vi "RemoveObject.vi"(8 "error in (no error)":errorcluster, 9 "Ancestor":string, 10 "Name":string, 11 "reference in":refnum<class "ViPER.lvclass">) -> (0 "error out":errorcluster, 3 "reference out":refnum<class "ViPER.lvclass">)   [LabVIEW 2022 SP3, in "ViPER.lvlib" / "ViPER.lvclass"]
doc: "### BSD License (http://www.opensource.org/licenses/bsd-license.php) Begin ###\n\nCopyright (c) 2018 Kurt Friday www.medulla.net\n\nAll rights reserved.\n\nRedistribution and use in source and binary forms, with or without\nmodification, are permitted provided that the following conditions are met:\n\n * Redistributions of source code must retain the above copyright\n notice, this list of conditions and the following disclaimer.\n\n * Redistributions in binary form must reproduce the above copyright\n notice, this list of conditions and the following disclaimer in the\n documentation and/or other materials provided with the distribution.\n\n * Neither the name of the <organization> nor the\n names of its contributors may be used to endorse or promote products\n derived from this software without specific prior written permission.\n\nTHIS SOFTWARE IS PROVIDED BY THE COPYRIGHT HOLDERS AND CONTRIBUTORS \"AS IS\" AND\nANY EXPRESS OR IMPLIED WARRANTIES, INCLUDING, BUT NOT LIMITED TO, THE IMPLIED\nWARRANTIES OF MERCHANTABILITY AND FITNESS FOR A PARTICULAR PURPOSE ARE\nDISCLAIMED. IN NO EVENT SHALL <COPYRIGHT HOLDER> BE LIABLE FOR ANY\nDIRECT, INDIRECT, INCIDENTAL, SPECIAL, EXEMPLARY, OR CONSEQUENTIAL DAMAGES\n(INCLUDING, BUT NOT LIMITED TO, PROCUREMENT OF SUBSTITUTE GOODS OR SERVICES;\nLOSS OF USE, DATA, OR PROFITS; OR BUSINESS INTERRUPTION) HOWEVER CAUSED AND\nON ANY THEORY OF LIABILITY, WHETHER IN CONTRACT, STRICT LIABILITY, OR TORT\n(INCLUDING NEGLIGENCE OR OTHERWISE) ARISING IN ANY WAY OUT OF THE USE OF THIS\nSOFTWARE, EVEN IF ADVISED OF THE POSSIBILITY OF SUCH DAMAGE."
uses:
  ViPER.lvclass
panel:
  # "### BSD License (http://www.opensource.org/licenses/bsd-license.php) Begin ###\n\nCopyright (c) 2018  Kurt Friday www.medulla.net\n\nAll rights reserved.\n\nRedistribution and use in source and binary forms, with or without\nmodification, are permitted provided that the following conditions are met:\n\n    * Redistributions of source code must retain the above copyright\n      notice, this list of conditions and the following disclaimer.\n\n    * Redistributions in binary form must reproduce the above copyright\n      notice, this list of conditions and the following disclaimer in the\n      documentation and/or other materials provided with the distribution.\n\n    * Neither the name of the <organization> nor the\n      names of its contributors may be used to endorse or promote products\n      derived from this software without specific prior written permission.\n\nTHIS SOFTWARE IS PROVIDED BY THE COPYRIGHT HOLDERS AND CONTRIBUTORS \"AS IS\" AND\nANY EXPRESS OR IMPLIED WARRANTIES, INCLUDING, BUT NOT LIMITED TO, THE IMPLIED\nWARRANTIES OF MERCHANTABILITY AND FITNESS FOR A PARTICULAR PURPOSE ARE\nDISCLAIMED. IN NO EVENT SHALL <COPYRIGHT HOLDER> BE LIABLE FOR ANY\nDIRECT, INDIRECT, INCIDENTAL, SPECIAL, EXEMPLARY, OR CONSEQUENTIAL DAMAGES\n(INCLUDING, BUT NOT LIMITED TO, PROCUREMENT OF SUBSTITUTE GOODS OR SERVICES;\nLOSS OF USE, DATA, OR PROFITS; OR BUSINESS INTERRUPTION) HOWEVER CAUSED AND\nON ANY THEORY OF LIABILITY, WHETHER IN CONTRACT, STRICT LIABILITY, OR TORT\n(INCLUDING NEGLIGENCE OR OTHERWISE) ARISING IN ANY WAY OUT OF THE USE OF THIS\nSOFTWARE, EVEN IF ADVISED OF THE POSSIBILITY OF SUCH DAMAGE."
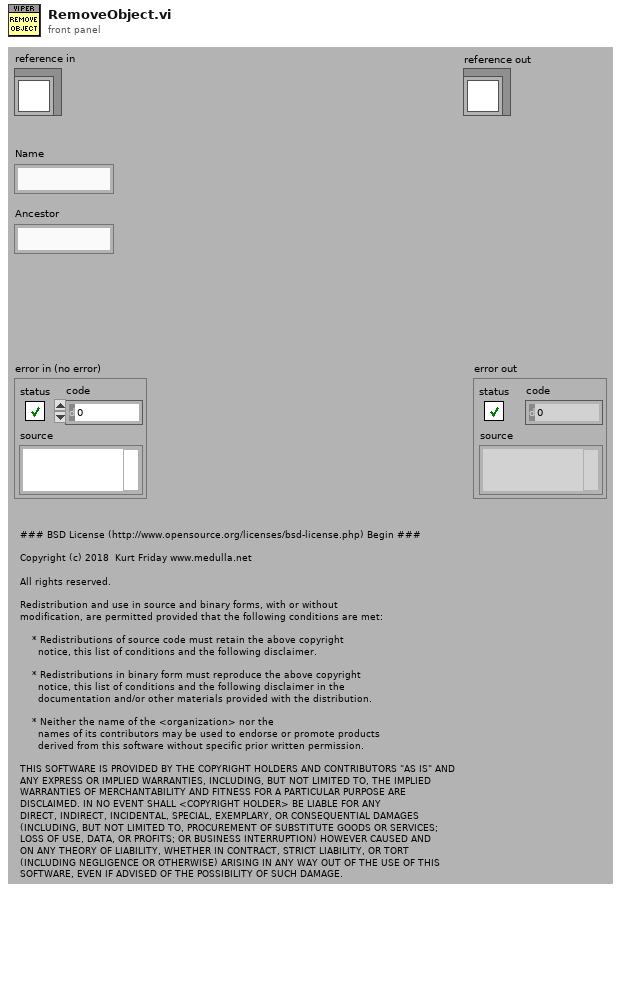
[diagram p1: front panel]
types:
  T1 = typedef "ViPER.lvlib/ViPER.lvclass/ObjectAttributes.ctl" = cluster{"Object":T2, "Ancestors":T4[], "Config":T5, "Init_OK":bool, "Hierachy":string[], "PPL?":bool[], "SFP_Open":bool[], "Config_SFP_Open":bool[], "SoftFP_event":refnum<user-event>[], "ConfigFP_event":refnum<user-event>[], "SoftFP_Shutdown_Notifier":refnum<notifier>[], "ConfigFP_Shutdown_Notifier":refnum<notifier>[]}
  T2 = typedef "ViPER.lvlib/ViPER.lvclass/ObjectDefinition.ctl" = cluster{"Name":string, "Ancestors":T3[]}
  T3 = typedef "ViPER.lvlib/ViPER.lvclass/Ancestor.ctl" = cluster{"Class":string, "Config":string, "Objects":string[]}
  T4 = typedef "ViPER.lvlib/ViPER.lvclass/ObjectLayers.ctl" = cluster{"Ancestor":string, "Objects":refnum<class "ViPER.lvclass">[], "Object_Names":string[], "Owned":bool[]}
  T5 = typedef "ViPER.lvlib/ViPER.lvclass/Config.ctl" = cluster{"default":string}
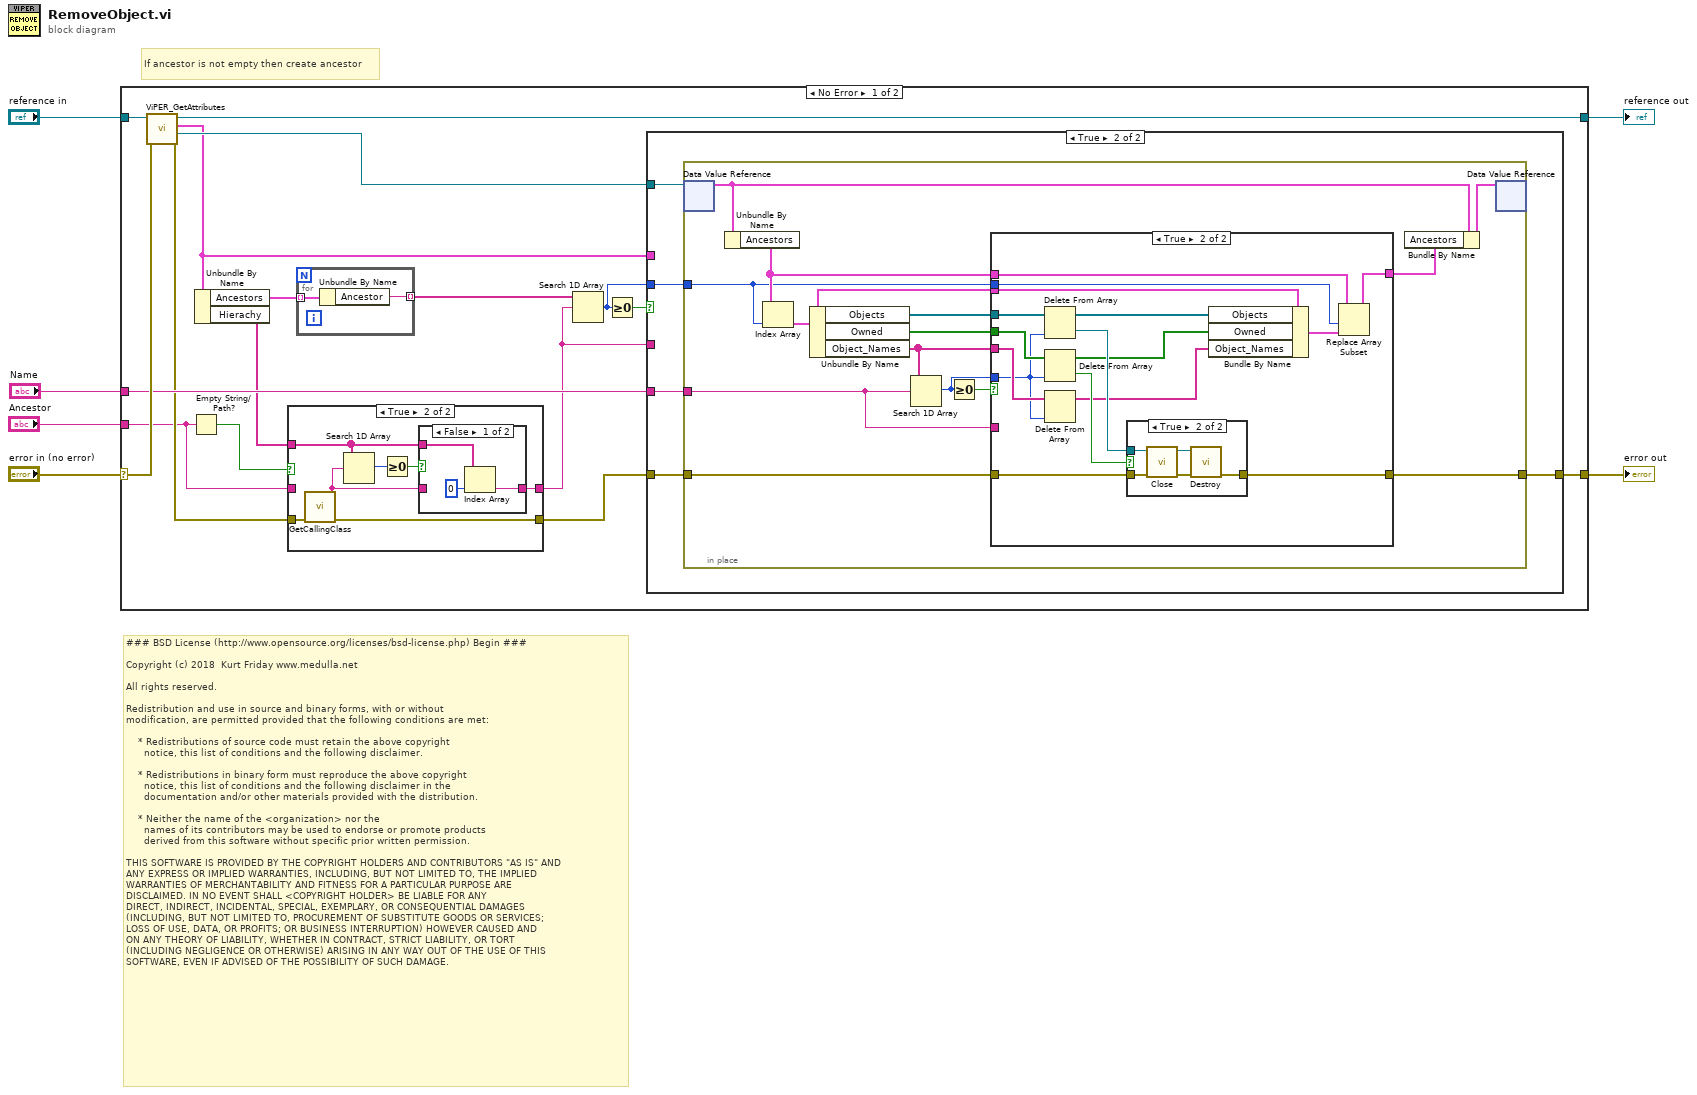
[diagram p0: block diagram]
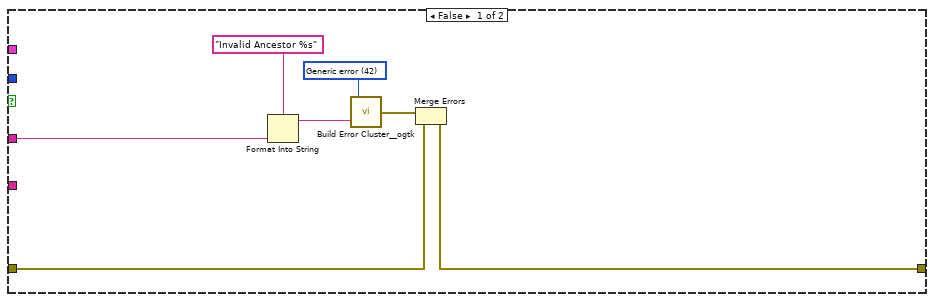
[diagram p4: hidden frame]
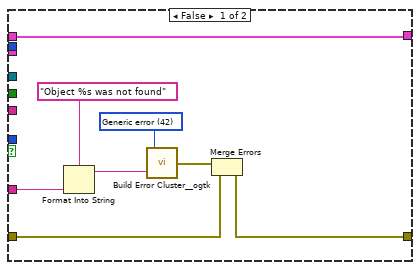
[diagram p5: hidden frame]
diagram:
  # "### BSD License (http://www.opensource.org/licenses/bsd-license.php) Begin ###\n\nCopyright (c) 2018  Kurt Friday www.medulla.net\n\nAll rights reserved.\n\nRedistribution and use in source and binary forms, with or without\nmodification, are permitted provided that the following conditions are met:\n\n    * Redistributions of source code must retain the above copyright\n      notice, this list of conditions and the following disclaimer.\n\n    * Redistributions in binary form must reproduce the above copyright\n      notice, this list of conditions and the following disclaimer in the\n      documentation and/or other materials provided with the distribution.\n\n    * Neither the name of the <organization> nor the\n      names of its contributors may be used to endorse or promote products\n      derived from this software without specific prior written permission.\n\nTHIS SOFTWARE IS PROVIDED BY THE COPYRIGHT HOLDERS AND CONTRIBUTORS \"AS IS\" AND\nANY EXPRESS OR IMPLIED WARRANTIES, INCLUDING, BUT NOT LIMITED TO, THE IMPLIED\nWARRANTIES OF MERCHANTABILITY AND FITNESS FOR A PARTICULAR PURPOSE ARE\nDISCLAIMED. IN NO EVENT SHALL <COPYRIGHT HOLDER> BE LIABLE FOR ANY\nDIRECT, INDIRECT, INCIDENTAL, SPECIAL, EXEMPLARY, OR CONSEQUENTIAL DAMAGES\n(INCLUDING, BUT NOT LIMITED TO, PROCUREMENT OF SUBSTITUTE GOODS OR SERVICES;\nLOSS OF USE, DATA, OR PROFITS; OR BUSINESS INTERRUPTION) HOWEVER CAUSED AND\nON ANY THEORY OF LIABILITY, WHETHER IN CONTRACT, STRICT LIABILITY, OR TORT\n(INCLUDING NEGLIGENCE OR OTHERWISE) ARISING IN ANY WAY OUT OF THE USE OF THIS\nSOFTWARE, EVEN IF ADVISED OF THE POSSIBILITY OF SUCH DAMAGE."
  # "If ancestor is not empty then create ancestor"
  n1 = case shown="No Error" "error in (no error)" {
    selector: "error in (no error)" -> [w21 w96]
    tunnel: [w17 w96] -> w5
    tunnel: [w22 w95] -> w3
    tunnel: "reference in" -> [w23 w95]
    tunnel: "Ancestor" -> [w9 _]
    tunnel: "Name" -> [w13 _]
    frame No Error {
      n2 = call "ViPER_GetAttributes.vi"("error in (no error)"=w21, "reference in"=w23) -> ("error out"=w12:errorcluster, "DataRef"=w15:refnum<data-value>, "Data"=w14:T1, "reference out"=w22:refnum<class "ViPER.lvclass">)  [unwired: 6 in]
      n3 = Empty String/Path?(string/path=w9) -> (empty?=w8:bool)
      n4 = Unbundle By Name(w14) -> ("Ancestors"=w20:T4[], "Hierachy"=w7:string[])
      n5 = case shown="True" w8 {
        tunnel: w12 -> [w24 w32]
        tunnel: [w24 w31] -> w11
        tunnel: [w25 w27] -> w10
        tunnel: w9 -> [w25 _]
        tunnel: w7 -> [_ w28]
        frame False {
        }
        frame True {
          n6 = call "GetCallingClass.vi"("error in (no error)"=w32) -> ("error out"=w31:errorcluster, "calling class"=w26:string)  [unwired: 9 in]
          n7 = Search 1D Array(1D array=w28, element=w26) -> (index of element=w30:i32)  [unwired: 1 in]
          n8 = Greater Or Equal To 0?(x=w30) -> (x >= 0?=w29:bool)
          n9 = case shown="False" w29 {
            tunnel: w28 -> [w35 _]
            tunnel: [w33 w36] -> w27
            tunnel: w26 -> [_ w36]
            frame False {
              n10 = Index Array(array=w35, index=0) -> (element=w33:string)
            }
            frame True {
            }
          }
        }
      }
      n11 = for {
        tunnel: w20 -> [w94] mode=indexing
        tunnel: [w93] -> w19 mode=indexing
        n12 = Unbundle By Name(w94) -> ("Ancestor"=w93:string)
      }
      n13 = Search 1D Array(1D array=w19, element=w10) -> (index of element=w16:i32)  [unwired: 1 in]
      n14 = Greater Or Equal To 0?(x=w16) -> (x >= 0?=w18:bool)
      n15 = case shown="True" w18 {
        tunnel: w11 -> [w39 w46]
        tunnel: [w38 w44] -> w17
        tunnel: w16 -> [_ w47]
        tunnel: w15 -> [_ w48]
        tunnel: w10 -> [w37 _]
        tunnel: w14 -> [_ _]
        tunnel: w13 -> [_ w45]
        frame False {
          w43 = 42 items=["No error", "Argument error", "Memory is full", "Out of zone", "End of file", "File already open", "Generic file I/O error", "File not found", "File permission error", "Disk is full", "Duplicate path", "Too many files open", "System feature not enabled", "Resource file not found", "Cannot add resource", "Resource not found", "Image not found", "Image memory error", "Pen does not exist", "Config type invalid", "Config token not found", "Config parse error", "Config memory error", "Bad external code format", "Bad external code offset", "External code not present", "Null window", "Destroy window error", "Null menu", "Print aborted", "Bad print record", "Print driver error", "Windows error during printing", "Memory error during printing", "Print dialog error", "Generic print error", "Invalid device refnum", "Device not found", "Device parameter error", "Device unit error", "Cannot open device", "Device call aborted", "Generic error", "Cancelled by user", "Object ID too low", "Object ID too high", "Object not in heap", "Unknown heap", "Unknown object (invalid DefProc)", "Unknown object (DefProc not in table)", "Message out of range", "Invalid (null) method", "Unknown message", "Manager call not supported", "Bad address", "Network operation in progress", "Network operation timed out", "Connection is busy", "Network attribute not supported", "Network error", "Address in use", "System out of memory", "Connection aborted", "Connection refused", "Not connected", "Already connected", "Connection closed", "Initialization error (interapplication manager)", "Bad occurrence", "Wait on unbound occurrence handler", "Occurrence queue overflow", "Datalog type conflict", "Unused", "Unrecognized type (interapplication manager)", "Memory corrupt", "Failed to make temporary DLL", "Old CIN version", "Drag socket not found", "Failed to load drop-object", "Failed to register OLE object", "Failed to release OLE object", "Format specifier type mismatch", "Unknown format specifier", "Too few format specifiers", "Too many format specifiers", "Scan failed", "Newer CIN version", "Error converting to variant", "Runtime menu error", "Password tampered", "Variant attribute not found", "Incompatible variant data type", "Event data is not available", "Event Store is not present", "Occurrence is not found", "Event Queue is not created", "Event info is not available", "Refnum passed is NULL", "Error retrieving Class GUID", "Error retrieving CoClass GUID", "Error retrieving TypeLib GUID.", "Bad built application magic bytes.", "Specific driver is different from the specific driver associated with the Logical Name.", "There is no session opened to the class driver.", "Max Error", "MAX - Error with config objects", "MAX - Error loading configuration", "MAX - Group not supported"]
          n16 = Format Into String(format string="Invalid Ancestor %s", w37) -> (resulting string=w40:string)  [unwired: 2 in, 1 out]
          n17 = call <userlib>:"Build Error Cluster__ogtk.vi"("String to Prepend to source (\"\")"=w40, "code"=w43) -> ("error out"=w42:errorcluster)
          n18 = Merge Errors(w42, w39) -> (w38:errorcluster)
        }
        frame True {
          n19 = in-place {
            in-place-border: w47 -> [w53]
            in-place-border: w46 -> [w51]
            in-place-border: w45 -> [w49]
            in-place-border: [w50] -> w44
            n20 = in-place-dvr #1(w48) -> (w61:T1)  [unwired: 1 out]
            n21 = Unbundle By Name(w61) -> ("Ancestors"=w60:T4[])
            n22 = Index Array(array=w60, index=w53) -> (element=w59:T4)
            n23 = Unbundle By Name(w59) -> ("Objects"=w54:refnum<class "ViPER.lvclass">[], "Owned"=w55:bool[], "Object_Names"=w56:string[])
            n24 = Search 1D Array(1D array=w56, element=w49) -> (index of element=w52:i32)  [unwired: 1 in]
            n25 = Greater Or Equal To 0?(x=w52) -> (x >= 0?=w57:bool)
            n26 = case shown="True" w57 {
              tunnel: w60 -> [w70 w86]
              tunnel: w59 -> [_ w85]
              tunnel: [w70 w83] -> w58
              tunnel: w56 -> [_ w78]
              tunnel: w55 -> [_ w79]
              tunnel: w54 -> [_ w81]
              tunnel: w53 -> [_ w82]
              tunnel: w52 -> [_ w77]
              tunnel: w51 -> [w67 w75]
              tunnel: [w66 w73] -> w50
              tunnel: w49 -> [w65 _]
              frame False {
                w69 = 42 items=["No error", "Argument error", "Memory is full", "Out of zone", "End of file", "File already open", "Generic file I/O error", "File not found", "File permission error", "Disk is full", "Duplicate path", "Too many files open", "System feature not enabled", "Resource file not found", "Cannot add resource", "Resource not found", "Image not found", "Image memory error", "Pen does not exist", "Config type invalid", "Config token not found", "Config parse error", "Config memory error", "Bad external code format", "Bad external code offset", "External code not present", "Null window", "Destroy window error", "Null menu", "Print aborted", "Bad print record", "Print driver error", "Windows error during printing", "Memory error during printing", "Print dialog error", "Generic print error", "Invalid device refnum", "Device not found", "Device parameter error", "Device unit error", "Cannot open device", "Device call aborted", "Generic error", "Cancelled by user", "Object ID too low", "Object ID too high", "Object not in heap", "Unknown heap", "Unknown object (invalid DefProc)", "Unknown object (DefProc not in table)", "Message out of range", "Invalid (null) method", "Unknown message", "Manager call not supported", "Bad address", "Network operation in progress", "Network operation timed out", "Connection is busy", "Network attribute not supported", "Network error", "Address in use", "System out of memory", "Connection aborted", "Connection refused", "Not connected", "Already connected", "Connection closed", "Initialization error (interapplication manager)", "Bad occurrence", "Wait on unbound occurrence handler", "Occurrence queue overflow", "Datalog type conflict", "Unused", "Unrecognized type (interapplication manager)", "Memory corrupt", "Failed to make temporary DLL", "Old CIN version", "Drag socket not found", "Failed to load drop-object", "Failed to register OLE object", "Failed to release OLE object", "Format specifier type mismatch", "Unknown format specifier", "Too few format specifiers", "Too many format specifiers", "Scan failed", "Newer CIN version", "Error converting to variant", "Runtime menu error", "Password tampered", "Variant attribute not found", "Incompatible variant data type", "Event data is not available", "Event Store is not present", "Occurrence is not found", "Event Queue is not created", "Event info is not available", "Refnum passed is NULL", "Error retrieving Class GUID", "Error retrieving CoClass GUID", "Error retrieving TypeLib GUID.", "Bad built application magic bytes.", "Specific driver is different from the specific driver associated with the Logical Name.", "There is no session opened to the class driver.", "Max Error", "MAX - Error with config objects", "MAX - Error loading configuration", "MAX - Group not supported"]
                n27 = Format Into String(format string="Object %s was not found", w65) -> (resulting string=w63:string)  [unwired: 2 in, 1 out]
                n28 = call <userlib>:"Build Error Cluster__ogtk.vi"("String to Prepend to source (\"\")"=w63, "code"=w69) -> ("error out"=w68:errorcluster)
                n29 = Merge Errors(w68, w67) -> (w66:errorcluster)
              }
              frame True {
                n30 = Delete From Array(array=w81, index=w77) -> (deleted portion=w74:refnum<class "ViPER.lvclass">, array with subset deleted=w80:refnum<class "ViPER.lvclass">[])  [unwired: 1 in]
                n31 = Delete From Array(array=w79, index=w77) -> (deleted portion=w76:bool, array with subset deleted=w72:bool[])  [unwired: 1 in]
                n32 = Delete From Array(array=w78, index=w77) -> (array with subset deleted=w71:string[])  [unwired: 1 in, 1 out]
                n33 = case shown="True" w76 {
                  tunnel: w75 -> [w87 w91]
                  tunnel: w74 -> [_ w92]
                  tunnel: [w87 w88] -> w73
                  frame False {
                  }
                  frame True {
                    n34 = call-dynamic "Close.vi"("error in (no error)"=w91, "reference in"=w92) -> ("error out"=w89:errorcluster, "reference out"=w90:refnum<class "ViPER.lvclass">)  [unwired: 8 in]
                    n35 = call "Destroy.vi"("error in (no error)"=w89, "reference in"=w90) -> ("error out"=w88:errorcluster)  [unwired: 9 in]
                  }
                }
                n36 = Bundle By Name(cluster=w85, "Objects"=w80, "Owned"=w72, "Object_Names"=w71) -> (w84:T4)
                n37 = Replace Array Subset(array=w86, new element=w84, index=w82) -> (w83:T4[])
              }
            }
            n38 = Bundle By Name(cluster=w61, "Ancestors"=w58) -> (w62:T1)
            n39 = in-place-dvr #1(w62) -> ()  [unwired: 2 out]
          }
        }
      }
    }
    frame Error {
    }
  }
  "error out" <- w5
  "reference out" <- w3
